vi "Get Service.vi"(7 "Service Type":refnum<class "Service.lvclass">, 8 "error in (no error)":errorcluster, 11 "Processing in":refnum<class "Processing.lvclass">) -> (0 "error out":errorcluster, 2 "Service":refnum<class "Service.lvclass">, 3 "Processing out":refnum<class "Processing.lvclass">)   [LabVIEW 2020, in "HTTP Server.lvlib" / "Processing.lvclass"]
uses:
  Processing.lvclass
  Processing.lvclass/Processing.ctl
  Values/Values.lvclass
  Service/Service.lvclass
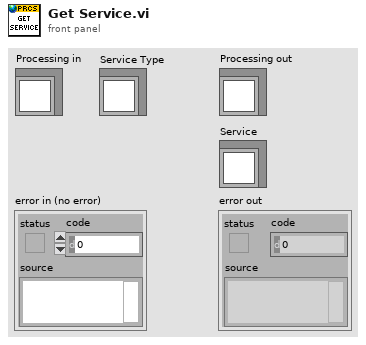
[diagram p1: front panel]
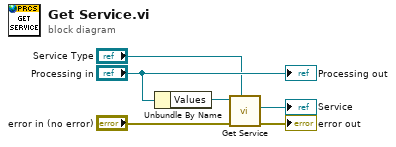
[diagram p0: block diagram]
diagram:
  n1 = Unbundle By Name("Processing in") -> ("Values"=w5:refnum<class "Values.lvclass">)
  n2 = call "Get Service.vi"("Service Type"="Service Type", "error in (no error)"="error in (no error)", "Values in"=w5) -> ("error out"=→"error out":errorcluster, "Service"=→"Service":refnum<class "Service.lvclass">)  [unwired: 6 in, 1 out]
  "Processing out" <- "Processing in"
